vi "PiColorWords.vi"(10 "String":string, 11 "String in":refnum<vi>) -> (3 "String out":refnum<vi>)   [LabVIEW 2019]
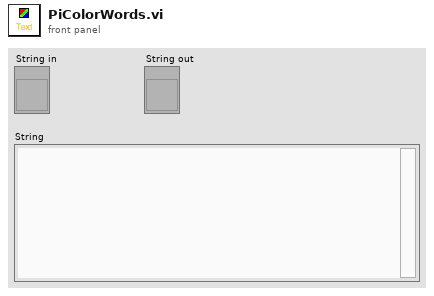
[diagram p1: front panel]
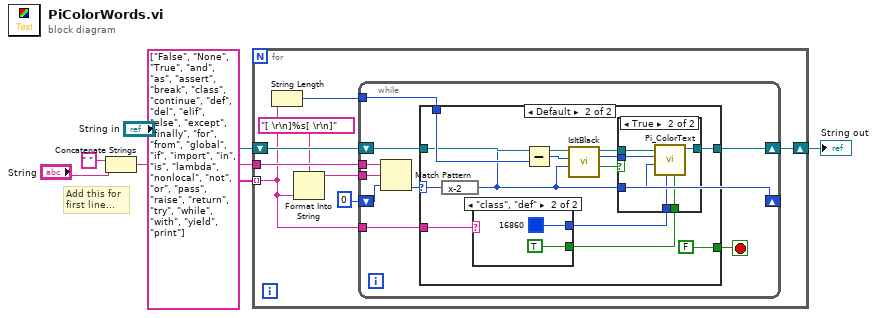
[diagram p0: block diagram]
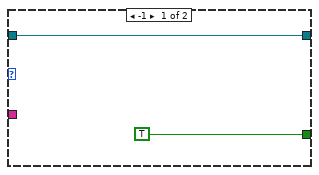
[diagram p2: hidden frame]
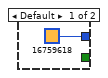
[diagram p4: hidden frame]
diagram:
  # "Add this for\nfirst line..."
  n1 = Concatenate Strings(" " ("string"), "String") -> (w1:string)
  n2 = for {
    shift-right: [w13] -> w6
    shift-left: "String in" -> [w14]
    tunnel: string[] ["False", "None", "True", "and", "as", "assert", "break", "class", "continue", "def", "del", "elif", "else", "except", "finally", "for", "from", "global", "if", "import", "in", "is", "lambda", "nonlocal", "not", "or", "pass", "raise", "return", "try", "while", "with", "yield", "print"] -> [w8] mode=indexing
    tunnel: w1 -> [w12]
    n3 = String Length(string=w8) -> (length=w7:i32)
    n4 = Format Into String(format string="[ \r\n]%s[ \r\n]" ("regular expression"), w8) -> (resulting string=w10:string)  [unwired: 2 in, 1 out]
    n5 = while {
      tunnel: w12 -> [w21]
      tunnel: w10 -> [w20]
      shift-right: [w22] -> w13
      shift-left: w14 -> [w23]
      shift-right: [w17] -> _
      shift-left: 0 -> [w18]
      tunnel: w7 -> [w16]
      tunnel: w8 -> [w15]
      stop <- w19 stop-if-true
      n6 = Match Pattern(string=w21, regular expression=w20, offset (0)=w18) -> (offset past match=w17:i32)  [unwired: 3 out]
      n7 = case shown="Default" w17 {
        selector: w17 -> [_ w31]
        tunnel: w23 -> [w24 w30]
        tunnel: [w24 w37] -> w22
        tunnel: [TRUE ("Text.Font:Bold") FALSE ("Text.Font:Bold")] -> w19
        tunnel: w16 -> [_ w35]
        tunnel: w15 -> [_ w33]
        frame -1 {
        }
        frame Default {
          n8 = expression code="x-2"(w31) -> (w26:i32)
          n9 = case shown="\"class\", \"def\"" w33 {
            tunnel: [u32 16759618 ("Text") u32 16860 ("Text")] -> w34
            tunnel: [_ TRUE ("Text.Font:Bold")] -> w32
            frame Default {
            }
            frame "class", "def" {
            }
          }
          n10 = Subtract(x=w26, y=w35) -> (x-y=w27:i32)
          n11 = call "IsItBlack.vi"("End"=w26, "Start"=w27, "String in"=w30) -> ("Black?"=w29:bool, "String out"=w28:refnum<vi>)  [unwired: 7 in]
          n12 = case shown="True" w29 {
            tunnel: [w38 w44] -> w37
            tunnel: w27 -> [_ w43]
            tunnel: w34 -> [_ w42]
            tunnel: w32 -> [_ w41]
            tunnel: w26 -> [_ w40]
            tunnel: w28 -> [w38 w39]
            frame False {
            }
            frame True {
              n13 = call "Pi_ColorText.vi"("Bold?"=w41, "Color"=w42, "End"=w40, "Start"=w43, "String in"=w39) -> ("String out"=w44:refnum<vi>)  [unwired: 6 in]
            }
          }
        }
      }
    }
  }
  "String out" <- w6
